vi "simple external error.vi"(8 "error in":errorcluster, 11 "cycle results":dbl[](array[numeric])) -> (0 "error out":errorcluster, 1 "percent error":dbl, 2 "External error":dbl, 3 "Sequence result":dbl format="%0.2f")   [LabVIEW 2016]
doc: "for simple error analysis, this takes the average value for each \ncycle in a sequence and gets the external error\nwhich is R(ext)^2=(1/(N*(N-1))*Sum(R-r(cycle)).\nWhere N is the number of cycles, R is the sequence ratio and r(cycle)\nis the cycle ratio"
uses:
  <vilib>/Analysis/baseanly.llb/Mean (DBL).vi
  <vilib>/Analysis/NI_AALBase.lvlib
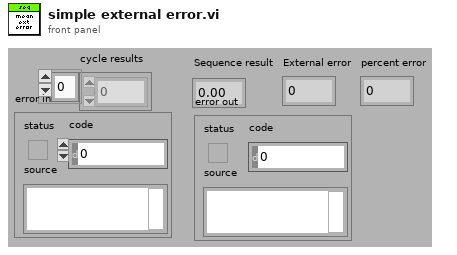
[diagram p1: front panel]
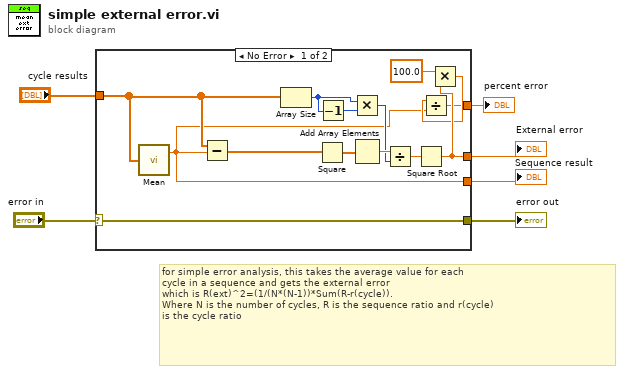
[diagram p0: block diagram]
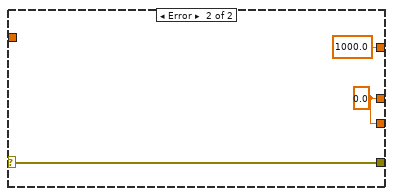
[diagram p2: hidden frame]
diagram:
  # "for simple error analysis, this takes the average value for each \ncycle in a sequence and gets the external error\nwhich is R(ext)^2=(1/(N*(N-1))*Sum(R-r(cycle)).\nWhere N is the number of cycles, R is the sequence ratio and r(cycle)\nis the cycle ratio"
  n1 = case shown="No Error" "error in" {
    selector: "error in" -> [w12 w22]
    tunnel: [w10 w23] -> w6
    tunnel: "cycle results" -> [w13 _]
    tunnel: [w8 w23] -> w4
    tunnel: [w12 w22] -> w2
    tunnel: [w7 1000.0] -> w1
    frame No Error {
      n2 = call-poly <vilib>:"Mean.vi"("X"=w13) -> ("mean"=w8:dbl)  [unwired: 1 out]
      n3 = Subtract(x=w13, y=w8) -> (x-y=w14:dbl[])
      n4 = Array Size(array=w13) -> (size(s)=w16:i32)
      n5 = Square(x=w14) -> (x^2=w19:dbl[])
      n6 = Decrement(x=w16) -> (x-1=w15:i32)
      n7 = Multiply(x=w16, y=w15) -> (x*y=w17:i32)
      n8 = Add Array Elements(numeric array=w19) -> (sum=w20:dbl)
      n9 = Divide(x=w20, y=w17) -> (x/y=w18:dbl)
      n10 = Square Root(x=w18) -> (sqrt(x)=w10:dbl)
      n11 = Multiply(x=100.0, y=w10) -> (x*y=w9:dbl)
      n12 = Divide(x=w9, y=w8) -> (x/y=w7:dbl)
    }
    frame Error {
      w23 = 0.0
    }
  }
  "External error" <- w6
  "Sequence result" <- w4
  "error out" <- w2
  "percent error" <- w1
